vi "cmd打开文件.vi"(8 "error in (no error)":errorcluster caption="错误输入（无错误）", 11 "文件路径":path) -> (0 "error out":errorcluster caption="错误输出")   [LabVIEW 2017]
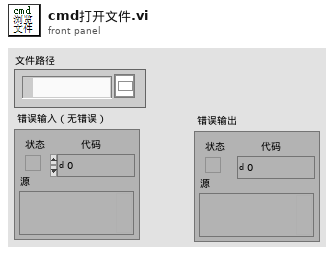
[diagram p1: front panel]
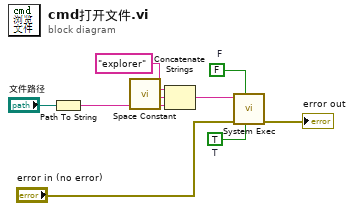
[diagram p0: block diagram]
diagram:
  w2 = FALSE  # F
  w9 = TRUE  # T
  n1 = Path To String(path="文件路径") -> (string=w7:string)
  n2 = call <vilib>:"Space Constant.vi"() -> ("String"=w6:string)
  n3 = Concatenate Strings("explorer", w6, w7) -> (w8:string)
  n4 = call <vilib>:"System Exec.vi"("run minimized? (F)"=w9, "wait until completion? (T)"=w2, "error in (no error)"="error in (no error)", "command line"=w8) -> ("error out"=→"error out":errorcluster)  [unwired: 4 in, 3 out]
